vi "Get Recoverable Network Streams Errors.vi"() -> (3 "recoverable network streams errors":i32[](array[numeric]))   [LabVIEW 2018]
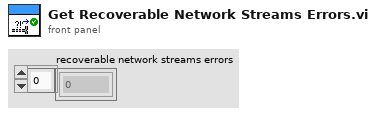
[diagram p1: front panel]
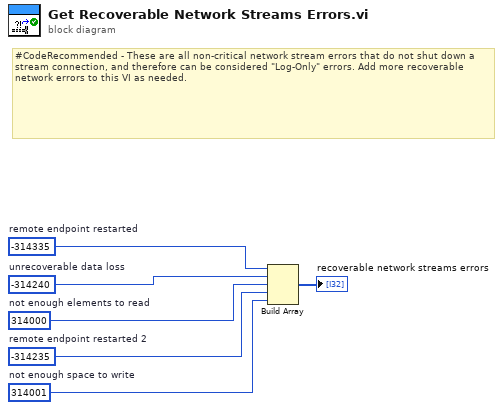
[diagram p0: block diagram]
diagram:
  w2 = 314001  # not enough space to write
  w4 = 314000  # not enough elements to read
  w3 = -314235  # remote endpoint restarted 2
  w5 = -314240  # unrecoverable data loss
  w6 = -314335  # remote endpoint restarted
  # "#CodeRecommended - These are all non-critical network stream errors that do not shut down a stream connection, and therefore can be considered \"Log-Only\" errors. Add more recoverable network errors to this VI as needed."
  n1 = Build Array(w6, w5, w4, w3, w2) -> (→"recoverable network streams errors":i32[])
